vi "calibrate polarizer newport.vi"() -> ()   [LabVIEW 2023, in "Power Meter.lvlib"]
uses:
  Power Meter.lvlib
  Thorlabs Polarizer/Thorlabs Polarizer.lvlib
  <vilib>/Instr/_visa.llb/VISA Configure Serial Port (Instr).vi
  C:/FlashGordon/Development/dll/ThorLabs.MotionControl.KCube.DCServoCLI.dll
  dll/ThorLabs.MotionControl.KCube.DCServoCLI.dll
panel:
  in  "Power meter COM port":refnum<visa-resource-name>
  out "Angles":dbl[](array[numeric])
  out "Angle":dbl
  out "Power":dbl
  in  "error in (no error)":errorcluster {"code" format="%.0x"}
  out "Power":dbl[](array[numeric])
  in  "Stop Button":bool
  out "error out":errorcluster
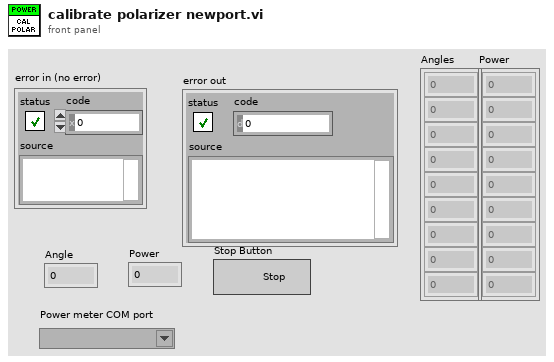
[diagram p1: front panel]
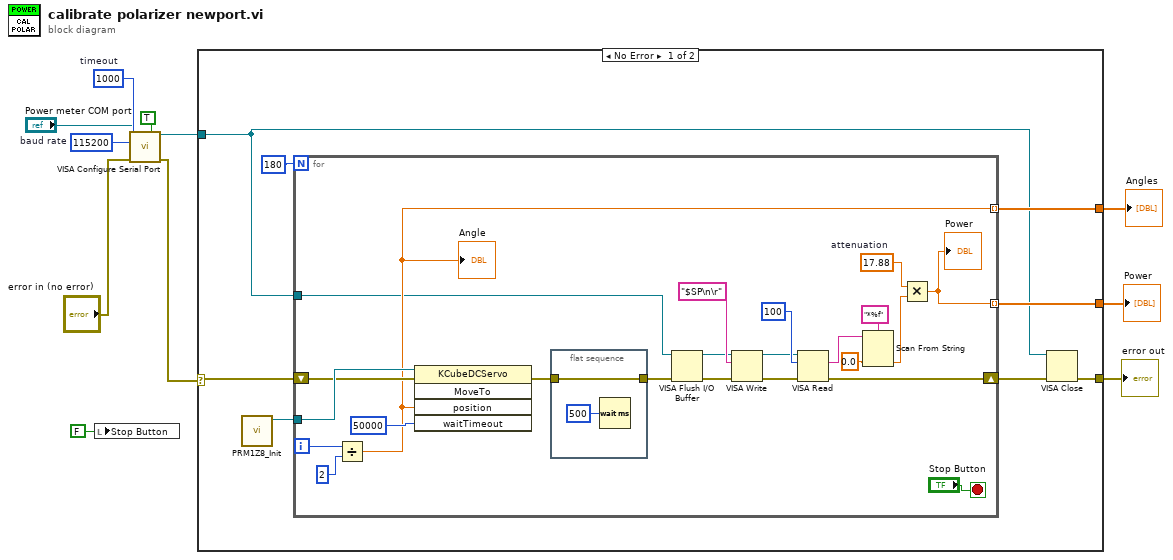
[diagram p0: block diagram]
diagram:
  w5 = u32 1000  # timeout
  w6 = u32 115200  # baud rate
  n1 = local write "Stop Button"(FALSE ("Stop Button")) -> ()
  n2 = call-poly "VISA Configure Serial Port"("VISA resource name"="Power meter COM port", "timeout (10sec)"=w5, "Enable Termination\nChar (T)"=TRUE ("Enable Termination\nChar (T)"), "baud rate (9600)"=w6, "error in (no error)"="error in (no error)") -> ("VISA resource name out"=w1:refnum<visa-resource-name>, "error out"=w2:errorcluster)  [unwired: 9 in]
  n3 = case shown="No Error" w2 {
    selector: w2 -> [w16 w45]
    tunnel: w1 -> [w12 _]
    tunnel: [w17 _] -> w11
    tunnel: [w13 w45] -> w10
    tunnel: [w15 _] -> w8
    frame No Error {
      n4 = call "PRM1Z8_Init.vi"() -> ("reference out"=w19:refnum<k24>)  [unwired: 10 in, 1 out]
      n5 = for {
        N: 180 -> [_]
        tunnel: w12 -> [w23]
        tunnel: [w35] -> w17 mode=indexing
        tunnel: w19 -> [w41]
        shift-right: [w21] -> w14
        shift-left: w16 -> [w40]
        tunnel: [w33] -> w15 mode=indexing
        i -> [w37]
        stop <- "Stop Button" stop-if-true
        w34 = 17.88  # attenuation
        n6 = Divide(x=w37, y=2) -> (x/y=w33:dbl)
        "Angle" <- w33
        n7 = invoke class="KCubeDCServo" method="MoveTo"(reference=w41, error in=w40, "position"=w33, "waitTimeout"=50000) -> (error out=w38:errorcluster)  [unwired: 1 in, 4 out]
        n8 = flat-sequence {
          tunnel: w38 -> [w44]
          tunnel: [w44] -> w22
          frame #0 {
            n9 = Wait (ms)(milliseconds to wait=u32 500) -> ()  [unwired: 1 out]
          }
        }
        n10 = VISA Flush I/O Buffer(VISA resource name=w23, error in (no error)=w22) -> (VISA resource name out=w30:refnum<visa-resource-name>, error out=w31:errorcluster)  [unwired: 1 in]
        n11 = VISA Write(VISA resource name=w30, write buffer="$SP\n\r", error in (no error)=w31) -> (VISA resource name out=w28:refnum<visa-resource-name>, error out=w27:errorcluster)  [unwired: 1 out]
        n12 = VISA Read(VISA resource name=w28, byte count=u32 100, error in (no error)=w27) -> (read buffer=w26:string, error out=w21:errorcluster)  [unwired: 2 out]
        n13 = Scan From String(format string="*%f", input string=w26, default 1=0.0 ("default value 1")) -> (output 1=w20:dbl)  [unwired: 2 in, 3 out]
        n14 = Multiply(x=w34, y=w20) -> (x*y=w35:dbl)
        "Power" <- w35
      }
      n15 = VISA Close(VISA resource name=w12, error in (no error)=w14) -> (error out=w13:errorcluster)
    }
    frame Error {
    }
  }
  "error out" <- w10
  "Power" <- w11
  "Angles" <- w8
